vi "Generic - DO1 - PULSE.vi"(0 "VISA session":refnum<visa-resource-name>="MW100", 2 "Semiphore":T1, 5 "Channel_Enum":T2=1 items=["4-20_OUT", "Pres_HI1", "Pres_HI2", "Pres_LOW", "Pres_PIN", "HEATER_TOP", "HEATER_BOT", "T_Shell", "FLOWMETER", "WATT_SENSE", "WH_TICK", "Tc_1", "Tc_2", "Tc_3", "Tc_4", "Tc_5", "Tc_6", "Tc_down", "T_Shell_2", "T_Shell_3", "T_Shell_4", "RTD_IN", "RTD_OUT", "RTD_AMB", "INTF_TEMPFLO", "INTF_READY", "INTF_START", "INTF_STOP", "DRM_LOW", "DRM_HIGH", "PWR_MAIN", "VLV_DUMP", "VLV_OUT", "VLV_IN", "WATT_HOURS", "FLOW(SAMPLE)", "GALLONS", "FLOW(GPM)", "FLOW_CALC_GAIN", "FLOW_CALC_OFFSET", "FLOW_CALC_THRESHOLD", "VLV_DUMP_2", "VLV_OUT_2", "VLV_IN_2", "VLV_DUMP_3", "VLV_OUT_3", "VLV_IN_3", "VLV_DUMP_4", "VLV_OUT_4", "VLV_IN_4", "CHAN_34", "CHAN_35", "CHAN_36"], 11 "Error In":errorcluster) -> (4 "dup VISA session":refnum<visa-resource-name>, 15 "error out":errorcluster)   [LabVIEW 2012]
uses:
  ChannelSettings.ctl
panel:
  in  "milliseconds to wait":u32=200
  out "Local?":bool
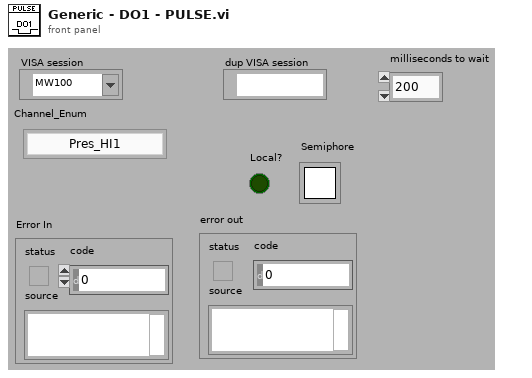
[diagram p1: front panel]
types:
  T1 = typedef "Semaphore RefNum" = refnum<k1>
  T2 = typedef "ChannelSettings.ctl" = u32
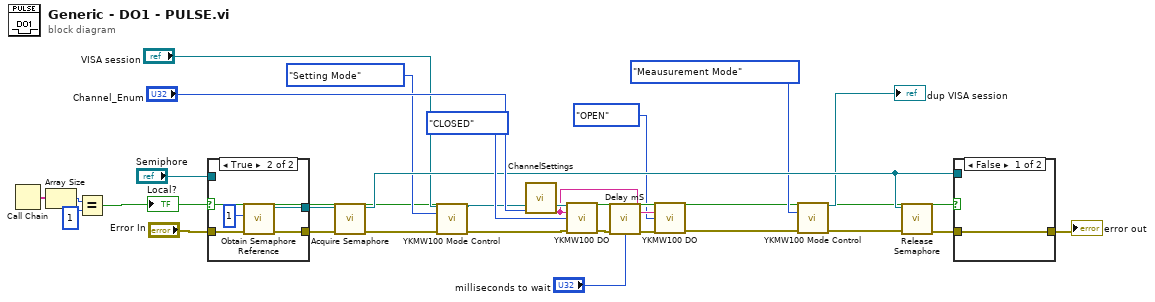
[diagram p0: block diagram]
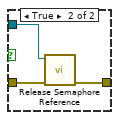
[diagram p2: hidden frame]
diagram:
  n1 = Call Chain() -> (call chain=w10:string[])
  n2 = Array Size(array=w10) -> (size(s)=w11:i32)
  n3 = Equal?(x=w11, y=1) -> (x = y?=w9:bool)
  "Local?" <- w9
  n4 = case shown="True" w9 {
    tunnel: [w30 w34] -> w27
    tunnel: "Error In" -> [w31 w33]
    tunnel: [w31 w32] -> w25
    tunnel: "Semiphore" -> [w30 _]
    frame False {
    }
    frame True {
      n5 = call <vilib>:"Obtain Semaphore Reference.vi"("error in (no error)"=w33, "size (1)"=1) -> ("error out"=w32:errorcluster, "semaphore"=w34:T1)  [unwired: 3 in, 1 out]
    }
  }
  n6 = call <vilib>:"Acquire Semaphore.vi"("error in (no error)"=w25, "semaphore"=w27) -> ("error out"=w20:errorcluster, "semaphore out"=w22:T1)  [unwired: 3 in, 1 out]
  n7 = call "YKMW100 Mode Control.vi"("VISA session"="VISA session", "Model"=enum16{"Meausurement Mode", "Setting Mode"}."Setting Mode", "error in (no error)"=w20) -> ("dup VISA session"=w18:refnum<visa-resource-name>, "error out"=w21:errorcluster)  [unwired: 11 in]
  n8 = call "ChannelSettings.vi"("Channel_Enum"="Channel_Enum") -> ("Channel String"=w6:string)  [unwired: 10 in]
  n9 = call "YKMW100 DO.vi"("VISA session"=w18, "P1 - Channel"=w6, "Relay Status (0:CLOSED)"=enum8{"CLOSED", "OPEN"}."CLOSED", "error in (no error)"=w21) -> ("dup VISA session"=w5:refnum<visa-resource-name>, "error out"=w8:errorcluster)  [unwired: 10 in]
  n10 = call "Delay mS.vi"("Error In"=w8, "milliseconds to wait"="milliseconds to wait") -> ("Error Out"=w7:errorcluster)  [unwired: 13 in]
  n11 = call "YKMW100 DO.vi"("VISA session"=w5, "P1 - Channel"=w6, "Relay Status (0:CLOSED)"=enum8{"CLOSED", "OPEN"}."OPEN", "error in (no error)"=w7) -> ("dup VISA session"=w2:refnum<visa-resource-name>, "error out"=w3:errorcluster)  [unwired: 10 in]
  n12 = call "YKMW100 Mode Control.vi"("VISA session"=w2, "Model"=enum16{"Meausurement Mode", "Setting Mode"}."Meausurement Mode", "error in (no error)"=w3) -> ("dup VISA session"=→"dup VISA session":refnum<visa-resource-name>, "error out"=w1:errorcluster)  [unwired: 11 in]
  n13 = call <vilib>:"Release Semaphore.vi"("error in (no error)"=w1, "semaphore"=w22) -> ("error out"=w24:errorcluster)  [unwired: 4 in, 1 out]
  n14 = case shown="False" w9 {
    tunnel: w24 -> [w36 w39]
    tunnel: [w36 w38] -> w23
    tunnel: w22 -> [_ w37]
    frame False {
    }
    frame True {
      n15 = call <vilib>:"Release Semaphore Reference.vi"("error in (no error)"=w39, "semaphore"=w37) -> ("error out"=w38:errorcluster)  [unwired: 8 in, 1 out]
    }
  }
  "error out" <- w23
